vi "PDash - Duplicate DQMH Module.vi"(4 "Original Tester":path, 6 "Original Library":path, 9 "New Tester":path, 10 "New Library":path, 11 "Project":refnum<vi>) -> (0 "error out":errorcluster)   [LabVIEW 2019]
doc: "_____\nCreated using DQMH Event Scripter 7.1.0.1447."
uses:
  PantherDashboard Scripting Hooks/Panther Dasboard Scripting Hooks.lvlib
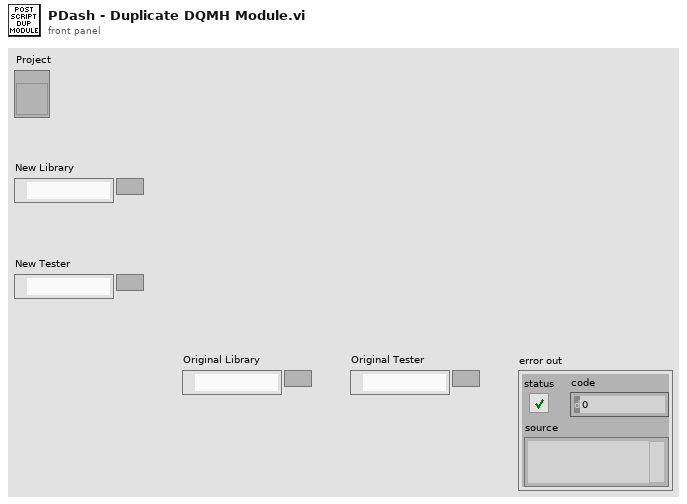
[diagram p1: front panel]
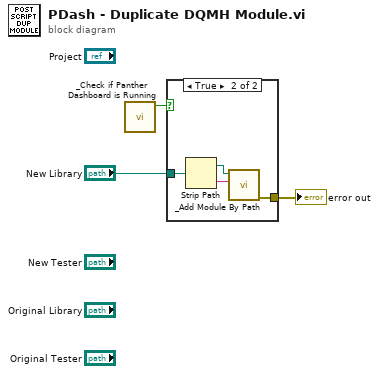
[diagram p0: block diagram]
diagram:
  n1 = call "_Check if Panther Dashboard is Running.vi"() -> ("Panther Dashboard is Running?"=w1:bool)  [unwired: 10 in, 1 out]
  n2 = case shown="True" w1 {
    tunnel: [_ w7] -> w3
    tunnel: "New Library" -> [_ w6]
    frame False {
    }
    frame True {
      n3 = Strip Path(path=w6) -> (stripped path=w5:path, name=w4:string)
      n4 = call "_Add Module By Path.vi"("New Module Name"=w4, "New Module Folder"=w5) -> ("error out"=w7:errorcluster)  [unwired: 9 in]
    }
  }
  "error out" <- w3
